vi "RecordErrorTime.vi"(8 "Error In":errorcluster) -> (0 "Error Out":errorcluster, 3 "current time":timestamp)   [LabVIEW 2018]
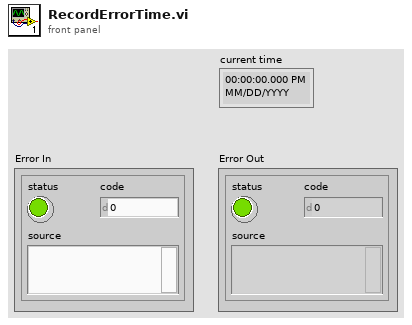
[diagram p1: front panel]
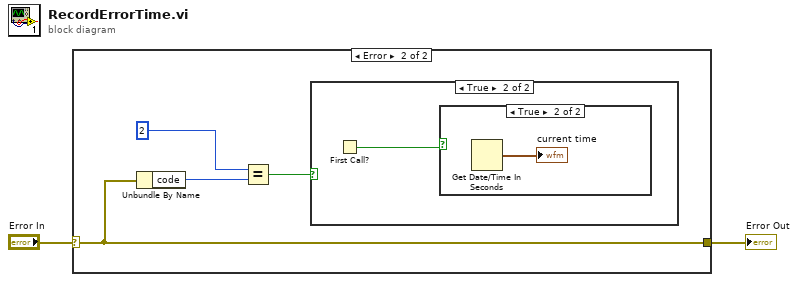
[diagram p0: block diagram]
diagram:
  n1 = case shown="Error" "Error In" {
    selector: "Error In" -> [w3 w7]
    tunnel: [w3 w7] -> w1
    frame No Error {
    }
    frame Error {
      n2 = Unbundle By Name(w7) -> ("code"=w6:i32)
      n3 = Equal?(x=2, y=w6) -> (x = y?=w4:bool)
      n4 = case shown="True" w4 {
        frame False {
        }
        frame True {
          n5 = First Call?() -> (First Call?: T/F=w8:bool)
          n6 = case shown="True" w8 {
            frame False {
            }
            frame True {
              n7 = Get Date/Time In Seconds() -> (seconds since 1Jan1904=→"current time":timestamp)
            }
          }
        }
      }
    }
  }
  "Error Out" <- w1
